vi "Property Tree Set Value_Select Items.vi"(8 "Error In":errorcluster, 9 "Tag Selected":string[](array[string]), 10 "Active Tree":refnum<vi>, 11 "All Tree Refs":refnum<vi>[](array[refnum])) -> (0 "Error Out":errorcluster)   [LabVIEW 2023]
doc: "Toggle has already happened, so here we determine if row is selecgted and deal with updating the tree value"
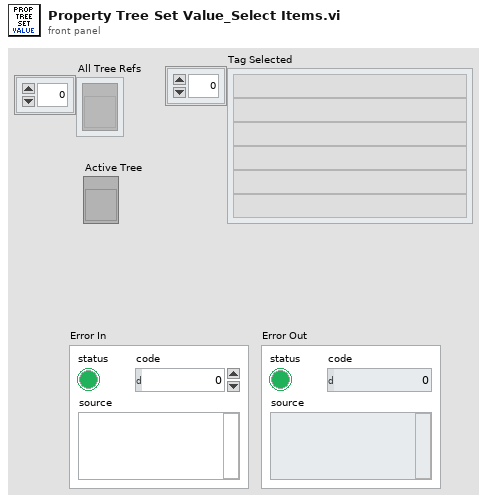
[diagram p1: front panel]
types:
  T1 = cluster{"Tag":string, "Read":bool, "Write":bool, "New":bool}
  T2 = enum16{"Init", "Read", "Remove", "Remove or Append", "Append", "Append If New"}
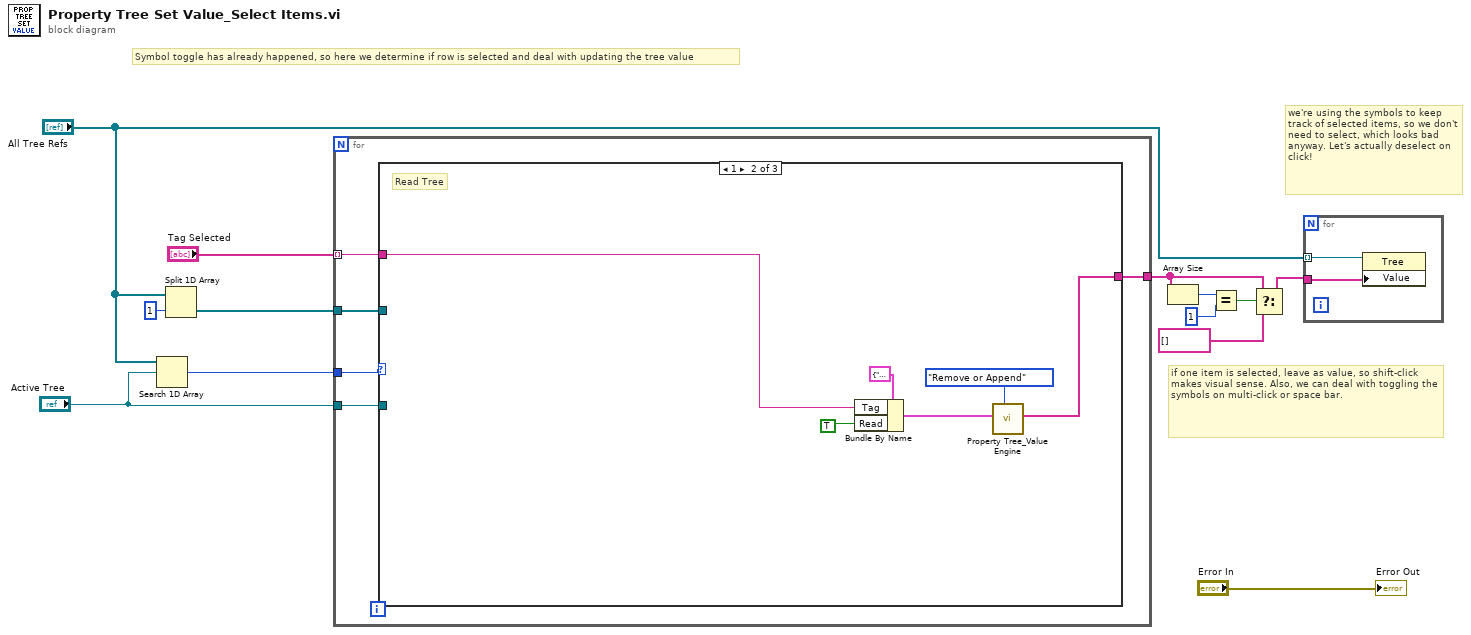
[diagram p0: block diagram]
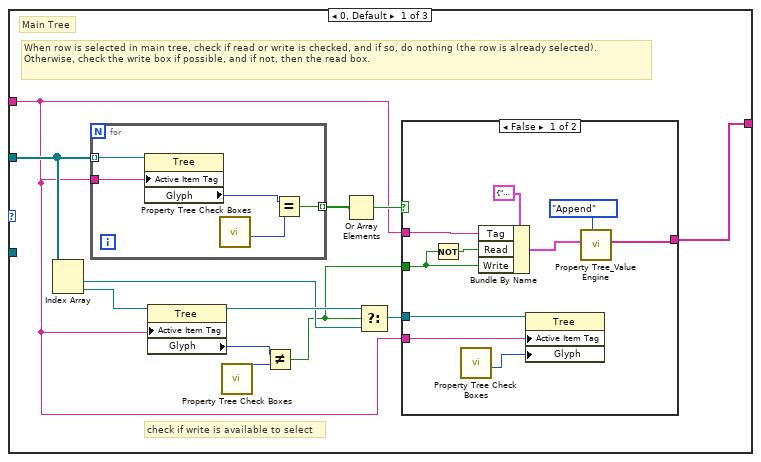
[diagram p2: hidden frame]
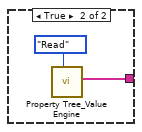
[diagram p3: hidden frame]
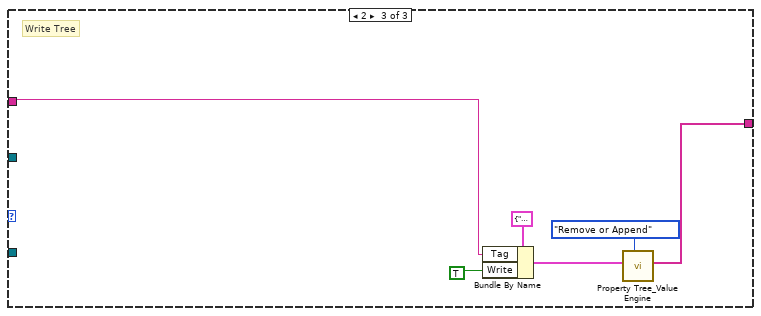
[diagram p4: hidden frame]
diagram:
  # "if one item is selected, leave as value, so shift-click makes visual sense. Also, we can deal with toggling the symbols on multi-click or space bar."
  # "we're using the symbols to keep track of selected items, so we don't need to select, which looks bad anyway. Let's actually deselect on click!"
  # "Symbol toggle has already happened, so here we determine if row is selected and deal with updating the tree value"
  n1 = Search 1D Array(1D array="All Tree Refs", element="Active Tree") -> (index of element=w13:i32)  [unwired: 1 in]
  n2 = Split 1D Array(array="All Tree Refs", index=1) -> (second subarray=w10:refnum<vi>[])  [unwired: 1 out]
  n3 = for {
    tunnel: w13 -> [w18]
    tunnel: "Active Tree" -> [w17]
    tunnel: w10 -> [w16]
    tunnel: "Tag Selected" -> [w15] mode=indexing
    tunnel: [w14] -> w3
    n4 = case shown="1" w18 {
      tunnel: w17 -> [_ _ _]
      tunnel: w16 -> [w29 _ _]
      tunnel: w15 -> [w19 w50 w56]
      tunnel: [w21 w51 w57] -> w14
      frame 0, Default {
        # "When row is selected in main tree, check if read or write is checked, and if so, do nothing (the row is already selected). Otherwise, check the write box if possible, and if not, then the read box."
        # "check if write is available to select"
        # "Main Tree"
        n5 = Index Array(array=w29) -> (element #1=w25:refnum<vi>, element #2=w27:refnum<vi>)  [unwired: 2 in]
        n6 = for {
          tunnel: w19 -> [w47]
          tunnel: w29 -> [w45] mode=indexing
          tunnel: [w44] -> w30 mode=indexing
          n7 = property class="Tree"(reference=w45, "Active Item Tag"=w47) -> ("Glyph"=w46:i32)  [unwired: 1 in, 2 out]
          n8 = call "Property Tree Check Boxes.vi"() -> ("Checked"=w43:i32)  [unwired: 9 in, 2 out]
          n9 = Equal?(x=w46, y=w43) -> (x = y?=w44:bool)
        }
        n10 = property class="Tree"(reference=w27, "Active Item Tag"=w19) -> (reference out=w26:refnum<vi>, "Glyph"=w28:i32)  [unwired: 1 in, 1 out]
        n11 = call "Property Tree Check Boxes.vi"() -> ("None"=w20:i32)  [unwired: 9 in, 2 out]
        n12 = Not Equal?(x=w28, y=w20) -> (x != y?=w22:bool)
        n13 = Or Array Elements(Boolean array=w30) -> (logical OR=w23:bool)
        n14 = Select(t=w26, s=w22, f=w25) -> (s? t:f=w24:refnum<vi>)
        n15 = case shown="False" w23 {
          tunnel: w24 -> [w40 _]
          tunnel: w19 -> [w38 _]
          tunnel: w22 -> [w36 _]
          tunnel: [w35 w42] -> w21
          tunnel: w19 -> [w34 _]
          frame False {
            n16 = Not(x=w36) -> (.not. x?=w37:bool)
            n17 = call "Property Tree Check Boxes.vi"() -> ("Checked"=w33:i32)  [unwired: 9 in, 2 out]
            n18 = Bundle By Name(cluster=T1 {"Tag"="", "Read"=FALSE, "Write"=FALSE, "New"=FALSE} ("Element"), "Tag"=w38, "Read"=w37, "Write"=w36) -> (w39:T1)
            n19 = property class="Tree"(reference=w40, "Active Item Tag"=w34, "Glyph"=w33) -> ()  [unwired: 1 in, 2 out]
            n20 = call "Property Tree_Value Engine.vi"("Save Action"=T2."Append" ("Action"), "Element"=w39) -> ("Tag Array"=w35:string[])  [unwired: 7 in, 2 out]
          }
          frame True {
            n21 = call "Property Tree_Value Engine.vi"("Save Action"=T2."Read" ("Action")) -> ("Tag Array"=w42:string[])  [unwired: 8 in, 2 out]
          }
        }
      }
      frame 1 {
        # "Read Tree"
        n22 = Bundle By Name(cluster=T1 {"Tag"="", "Read"=FALSE, "Write"=FALSE, "New"=FALSE} ("Element"), "Tag"=w50, "Read"=TRUE) -> (w53:T1)
        n23 = call "Property Tree_Value Engine.vi"("Save Action"=T2."Remove or Append" ("Action"), "Element"=w53) -> ("Tag Array"=w51:string[])  [unwired: 7 in, 2 out]
      }
      frame 2 {
        # "Write Tree"
        n24 = Bundle By Name(cluster=T1 {"Tag"="", "Read"=FALSE, "Write"=FALSE, "New"=FALSE} ("Element"), "Tag"=w56, "Write"=TRUE) -> (w59:T1)
        n25 = call "Property Tree_Value Engine.vi"("Save Action"=T2."Remove or Append" ("Action"), "Element"=w59) -> ("Tag Array"=w57:string[])  [unwired: 7 in, 2 out]
      }
    }
  }
  n26 = Array Size(array=w3) -> (size(s)=w6:i32)
  n27 = Equal?(x=w6, y=1) -> (x = y?=w4:bool)
  n28 = Select(t=w3, s=w4, f=string[] [] ("Tag Array")) -> (s? t:f=w2:string[])
  n29 = for {
    tunnel: w2 -> [w60]
    tunnel: "All Tree Refs" -> [w61] mode=indexing
    n30 = property class="Tree"(reference=w61, "Value"=w60) -> ()  [unwired: 1 in, 2 out]
  }
  "Error Out" <- "Error In"
